vi "SBE Clear Errors.vi"(7 "Enable (yes:TRUE)":bool=TRUE, 8 "error in (no error)":errorcluster, 9 "Clear all (No: FALSE)":bool, 10 "Error Codes Array":i32[](array[numeric]), 11 "Error Code":i32) -> (0 "error out":errorcluster, 3 "Cleared?":bool)   [LabVIEW 2017]
doc: "Clears incoming errors.\n\nClears the incoming error if the error code matches the value of <B>Error Code</B> or the values in the <B>Error Codes</B> Array and enable is TRUE. Clears any error if <B>Clear all</B> is true. The error cluster is passed through if the status boolean is false or if no match is found.\n<B>Copyright © 2004 Saint Bernard Engineering, Inc.</B>"
panel:
  # "Copyright © 2004 Saint Bernard Engineering, Inc."
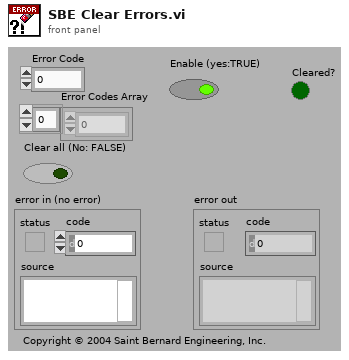
[diagram p1: front panel]
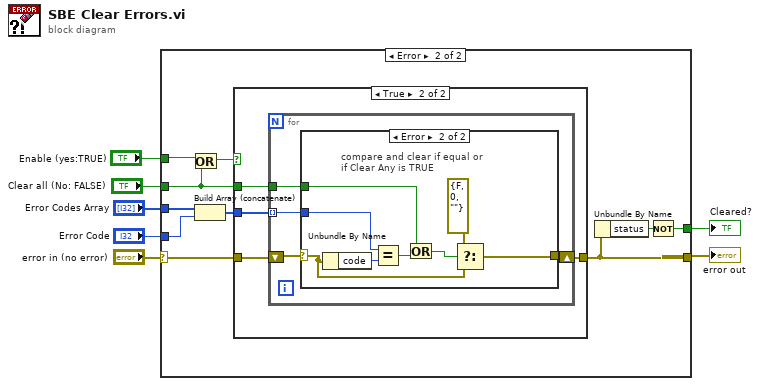
[diagram p0: block diagram]
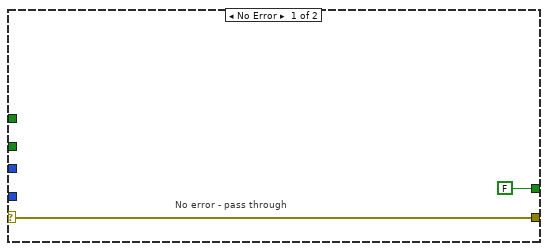
[diagram p2: hidden frame]
diagram:
  n1 = case shown="Error" "error in (no error)" {
    selector: "error in (no error)" -> [w9 w13]
    tunnel: [w9 w12] -> w6
    tunnel: "Error Code" -> [_ w18]
    tunnel: "Error Codes Array" -> [_ w19]
    tunnel: "Clear all (No: FALSE)" -> [_ w15]
    tunnel: "Enable (yes:TRUE)" -> [_ w16]
    tunnel: [FALSE w10] -> w1
    frame No Error {
      # "No error - pass through"
    }
    frame Error {
      n2 = Or(x=w16, y=w15) -> (x .or. y?=w14:bool)
      n3 = Build Array (concatenate)(w19, w18) -> (w17:i32[])
      n4 = case shown="True" w14 {
        tunnel: w13 -> [w20 w24]
        tunnel: w17 -> [_ w23]
        tunnel: [w20 w22] -> w12
        tunnel: w15 -> [_ w21]
        frame False {
        }
        frame True {
          n5 = for {
            shift-right: [w26] -> w22
            shift-left: w24 -> [w28]
            tunnel: w23 -> [w27] mode=indexing
            tunnel: w21 -> [w25]
            n6 = case shown="Error" w28 {
              selector: w28 -> [w29 w33]
              tunnel: w27 -> [_ w35]
              tunnel: [w29 w34] -> w26
              tunnel: w25 -> [_ w32]
              frame No Error {
                # "Error has been cleared. Pass cleared\nerror cluster through"
              }
              frame Error {
                # "compare and clear if equal or \nif Clear Any is TRUE"
                n7 = Unbundle By Name(w33) -> ("code"=w36:i32)
                n8 = Equal?(x=w35, y=w36) -> (x = y?=w30:bool)
                n9 = Or(x=w32, y=w30) -> (x .or. y?=w31:bool)
                n10 = Select(t=errorcluster {"status"=FALSE, "code"=0, "source"=""}, s=w31, f=w33) -> (s? t:f=w34:errorcluster)
              }
            }
          }
        }
      }
      n11 = Unbundle By Name(w12) -> ("status"=w11:bool)
      n12 = Not(x=w11) -> (.not. x?=w10:bool)
    }
  }
  "error out" <- w6
  "Cleared?" <- w1
